vi "Configure Adapter Removal.vi"(7 "Adapter Length (0.0)":dbl format="%.2f", 8 "error in (no error)":errorcluster, 9 "Port 1 (1)":i32=1, 10 "Channel (1)":i32=1, 11 "VISA resource name":refnum<visa-resource-name>) -> (0 "error out":errorcluster, 3 "VISA resource name out":refnum<visa-resource-name>)   [LabVIEW 2020, in "Agilent ENA Series.lvlib"]
doc: "Configures Adapter Removal.\n\nNotes:\n(1) Only E5063A, E5071C and E5072A supports this function.\n(2) Not supported by the E5070B, E5071B, E5061B, E5061A, E5062A, E5080A and E5080B"
uses:
  <instrlib>/Agilent ENA Series/Agilent ENA Series.lvlib
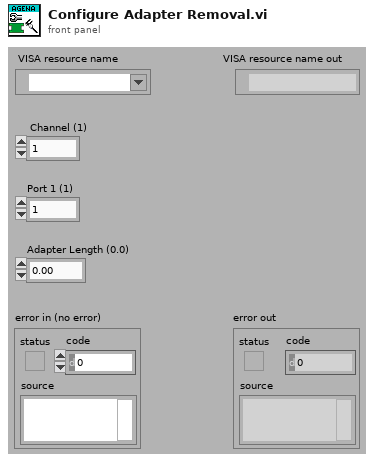
[diagram p1: front panel]
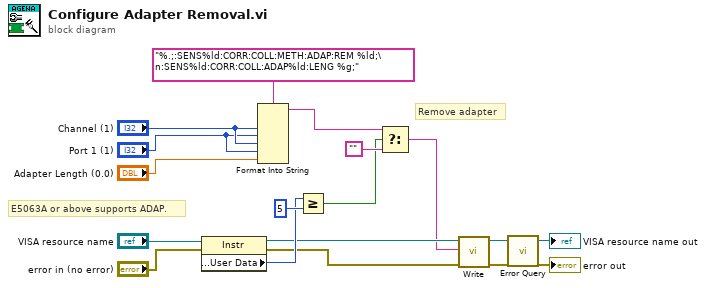
[diagram p0: block diagram]
diagram:
  # "E5063A or above supports ADAP."
  # "Remove adapter"
  n1 = property on="Property Node" class="Instr"(reference="VISA resource name", error in="error in (no error)") -> (reference out=w7:refnum<visa-resource-name>, error out=w5:errorcluster, "General Settings:User Data"=w14:u32)
  n2 = Format Into String(format string="%.;:SENS%ld:CORR:COLL:METH:ADAP:REM %ld;\n:SENS%ld:CORR:COLL:ADAP%ld:LENG %g;", "Channel (1)", "Port 1 (1)", "Channel (1)", "Port 1 (1)", "Adapter Length (0.0)") -> (resulting string=w8:string)  [unwired: 2 in, 1 out]
  n3 = Greater Or Equal?(x=w14, y=u32 5) -> (x >= y?=w13:bool)
  n4 = Select(t=w8, s=w13, f="") -> (s? t:f=w6:string)
  n5 = call <instrlib>:"Write.vi"("error in (no error)"=w5, "String ()"=w6, "VISA resource name"=w7) -> ("error out"=w3:errorcluster, "VISA resource name out"=w4:refnum<visa-resource-name>)  [unwired: 6 in, 1 out]
  n6 = call <instrlib>:"Error Query.vi"("error in (no error)"=w3, "VISA resource name"=w4) -> ("error out"=→"error out":errorcluster, "VISA resource name out"=→"VISA resource name out":refnum<visa-resource-name>)  [unwired: 6 in, 2 out]
